vi "SwerveJoystickRotationScaling.vi"(5 "Rotation Maximum":dbl(slide)=1.0 min=0.3 max=1.0 scale=0.3..1.0, 7 "Rotation Scaling":dbl(slide)=2.0 min=1.0 max=4.0 scale=1.0..4.0, 8 "Rotation Deadband":dbl(slide)=0.05 min=0.0 max=0.25 scale=0.0..0.25, 9 "Auto Control":bool, 10 "Raw Joystick Rotation":dbl) -> (0 "Scaled Joystick Rotation":dbl format="%.2f", 2 "In Deadband":bool)   [LabVIEW 2020]
doc: "Applies a deadband and nonlinear scaling to the rotation axis of a swerve drive. Includes a hook to override the non-linear deadband and scaling when the rotation is under autonomous control."
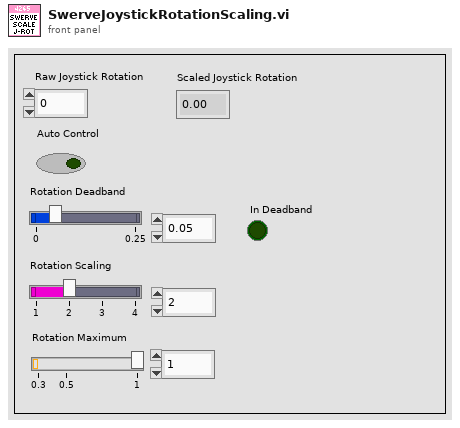
[diagram p1: front panel]
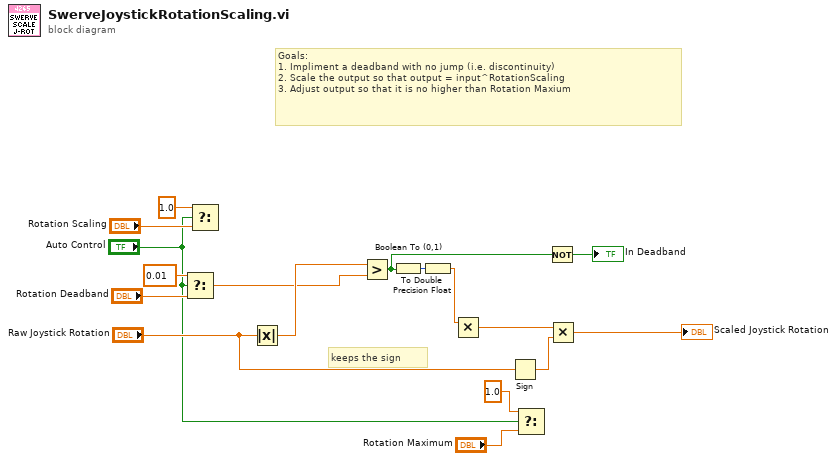
[diagram p0: block diagram]
diagram:
  # "keeps the sign"
  # "Goals:\n1. Impliment a deadband with no jump (i.e. discontinuity)\n2. Scale the output so that output = input^RotationScaling\n3. Adjust output so that it is no higher than Rotation Maxium"
  n1 = Select(t=0.01, s="Auto Control", f="Rotation Deadband") -> (s? t:f=w8:dbl)
  n2 = Select(t=1.0, s="Auto Control", f="Rotation Scaling") -> ()  [unwired: 1 out]
  n3 = Absolute Value(x="Raw Joystick Rotation") -> (abs(x)=w15:dbl)
  n4 = Greater?(x=w15, y=w8) -> (0:w16:bool)
  n5 = Boolean To (0,1)(Boolean=w16) -> (0, 1=w12:i16)
  n6 = To Double Precision Float(number=w12) -> (double precision float=w13:dbl)
  n7 = Multiply(x=w13) -> (x*y=w2:dbl)  [unwired: 1 in]
  n8 = Sign(1:"Raw Joystick Rotation") -> (0:w14:dbl)
  n9 = Select(t=1.0, s="Auto Control", f="Rotation Maximum") -> ()  [unwired: 1 out]
  n10 = Not(x=w16) -> (.not. x?=→"In Deadband":bool)
  n11 = Multiply(x=w2, y=w14) -> (x*y=→"Scaled Joystick Rotation":dbl)
